vi "Ctor.vi"(8 "error in (no error)":errorcluster) -> (0 "error out":errorcluster, 3 "Security out":refnum<class "Security.lvclass">)   [LabVIEW 2020, in "HTTP Server.lvlib" / "Security.lvclass"]
uses:
  Security.lvclass
  Security.lvclass/Security.ctl
  Ref Data.ctl
  Hierarchy.ctl
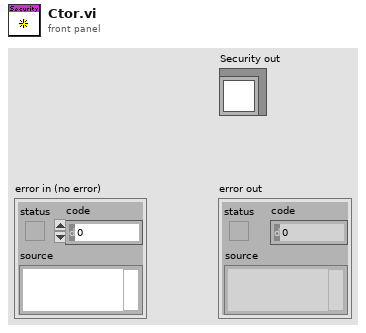
[diagram p1: front panel]
types:
  T1 = typedef "HTTP Server.lvlib/Security.lvclass/Ref Data.ctl" = cluster{"Hierarchy":T2}
  T2 = typedef "HTTP Server.lvlib/Security.lvclass/Hierarchy.ctl" = map{string, set{string}}
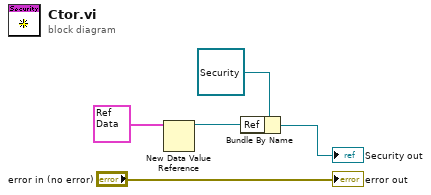
[diagram p0: block diagram]
diagram:
  n1 = New Data Value Reference(data value=T1 {"Hierarchy"={}} ("Ref Data")) -> (data value reference=w1:refnum<data-value>)  [unwired: 1 in, 1 out]
  n2 = Bundle By Name(cluster=refnum<class "Security.lvclass"> refnum ("Security in"), "Ref"=w1) -> (→"Security out":refnum<class "Security.lvclass">)
  "error out" <- "error in (no error)"
